vi "Write Data.vi"(10 "Data":i32, 11 "Linear Actuator Control Task Msg in":refnum<class "Linear Actuator Control Task Msg.lvclass">) -> (3 "Linear Actuator Control Task Msg out":refnum<class "Linear Actuator Control Task Msg.lvclass">)   [LabVIEW 2018, in "Linear Actuator Control Actor.lvlib" / "Linear Actuator Control Task Msg.lvclass"]
uses:
  Linear Actuator Control Task Msg.lvclass
  Linear Actuator Control Task Msg.lvclass/Linear Actuator Control Task Msg.ctl
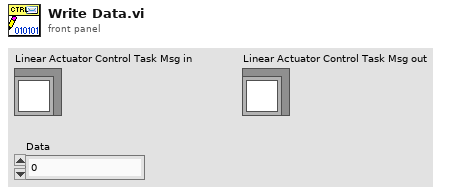
[diagram p1: front panel]
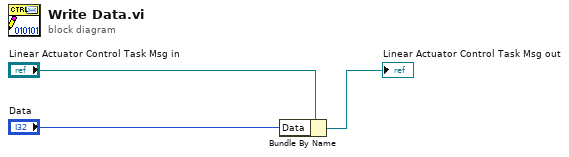
[diagram p0: block diagram]
diagram:
  n1 = Bundle By Name(cluster="Linear Actuator Control Task Msg in", "Data"="Data") -> (→"Linear Actuator Control Task Msg out":refnum<class "Linear Actuator Control Task Msg.lvclass">)
